vi "Write HTS dU.vi"(8 "error in (no error)":errorcluster, 10 "HTS dU":dbl, 11 "HTS Results in":refnum<class "HTS Results.lvclass">) -> (0 "error out":errorcluster, 3 "HTS Results out":refnum<class "HTS Results.lvclass">)   [LabVIEW 2019, in "Results.lvlib" / "HTS Results.lvclass"]
uses:
  HTS Results.lvclass
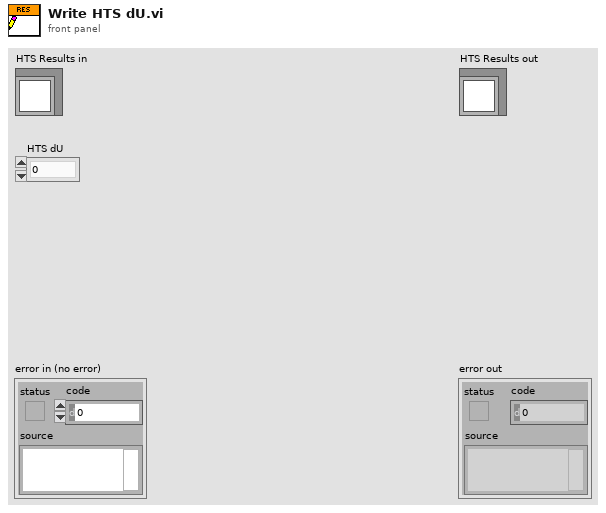
[diagram p1: front panel]
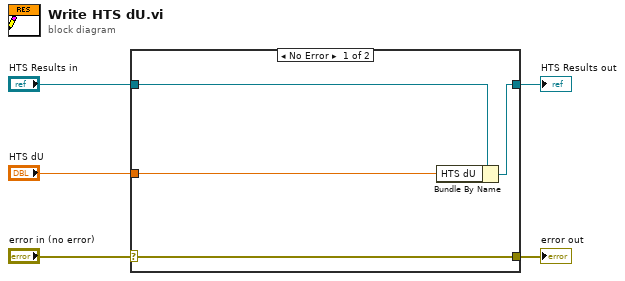
[diagram p0: block diagram]
diagram:
  n1 = case shown="No Error" "error in (no error)" {
    selector: "error in (no error)" -> [w9 w10]
    tunnel: [w9 w10] -> w4
    tunnel: [w7 w11] -> w2
    tunnel: "HTS Results in" -> [w8 w11]
    tunnel: "HTS dU" -> [w6 _]
    frame No Error {
      n2 = Bundle By Name(cluster=w8, "HTS dU"=w6) -> (w7:refnum<class "HTS Results.lvclass">)
    }
    frame Error {
    }
  }
  "error out" <- w4
  "HTS Results out" <- w2
